vi "Rx-Maping Detail's.vi"(7 "Data Cluster In":T1, 8 "error in (no error)":errorcluster) -> (0 "error out":errorcluster, 5 "Data Cluster Out":T1)   [LabVIEW 2021, in "Test Panel.lvlib"]
doc: "<b>Note:</b> This VI was modified by the <b>Validate DQMH Module</b> tool to turn off automatic error handling."
uses:
  Test Panel.lvlib
  Module Data--cluster.ctl
  GUI Ctrl Data's--Cluster.ctl
  Rx-Mapping Data.ctl
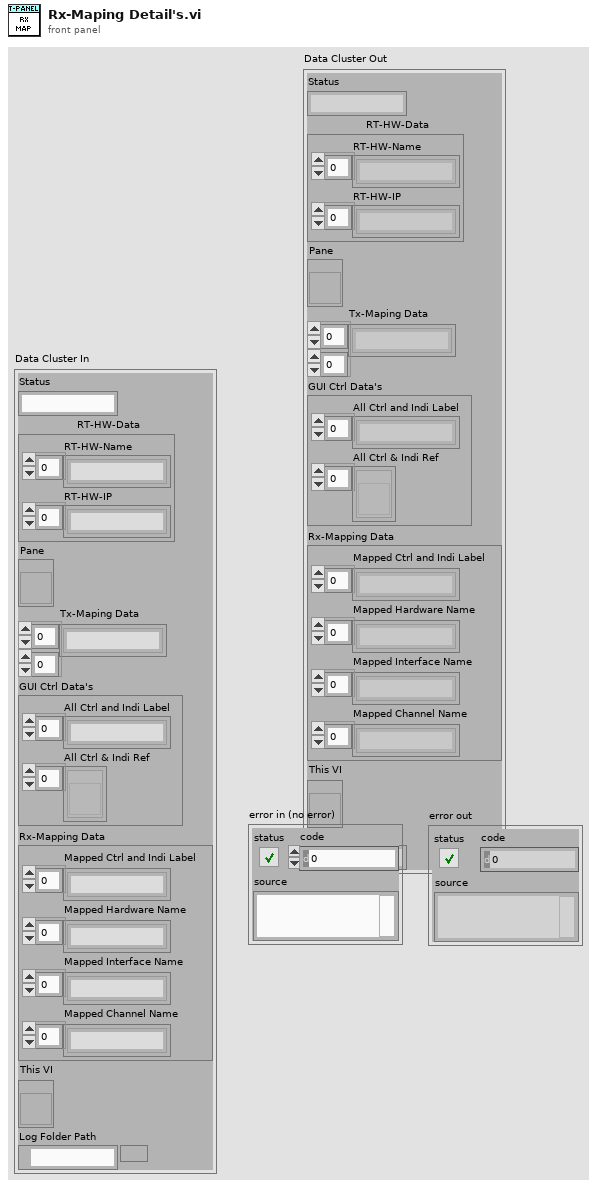
[diagram p1: front panel]
types:
  T1 = typedef "Test Panel.lvlib/Module Data--cluster.ctl" = cluster{"Status":string, "RT-HW-Data":cluster{"RT-HW-Name":string[], "RT-HW-IP":string[]}, "Pane":refnum<vi>, "Tx-Maping Data":string[][], "GUI Ctrl Data's":T2, "Rx-Mapping Data":T3, "This VI":refnum<vi>, "Log Folder Path":path}
  T2 = typedef "Test Panel.lvlib/GUI Ctrl Data's--Cluster.ctl" = cluster{"All Ctrl and Indi Label":string[], "All Ctrl & Indi Ref":refnum<vi>[]}
  T3 = typedef "Test Panel.lvlib/Rx-Mapping Data.ctl" = cluster{"Mapped Ctrl and Indi Label":string[], "Mapped Hardware Name":string[], "Mapped Interface Name":string[], "Mapped Channel Name":string[]}
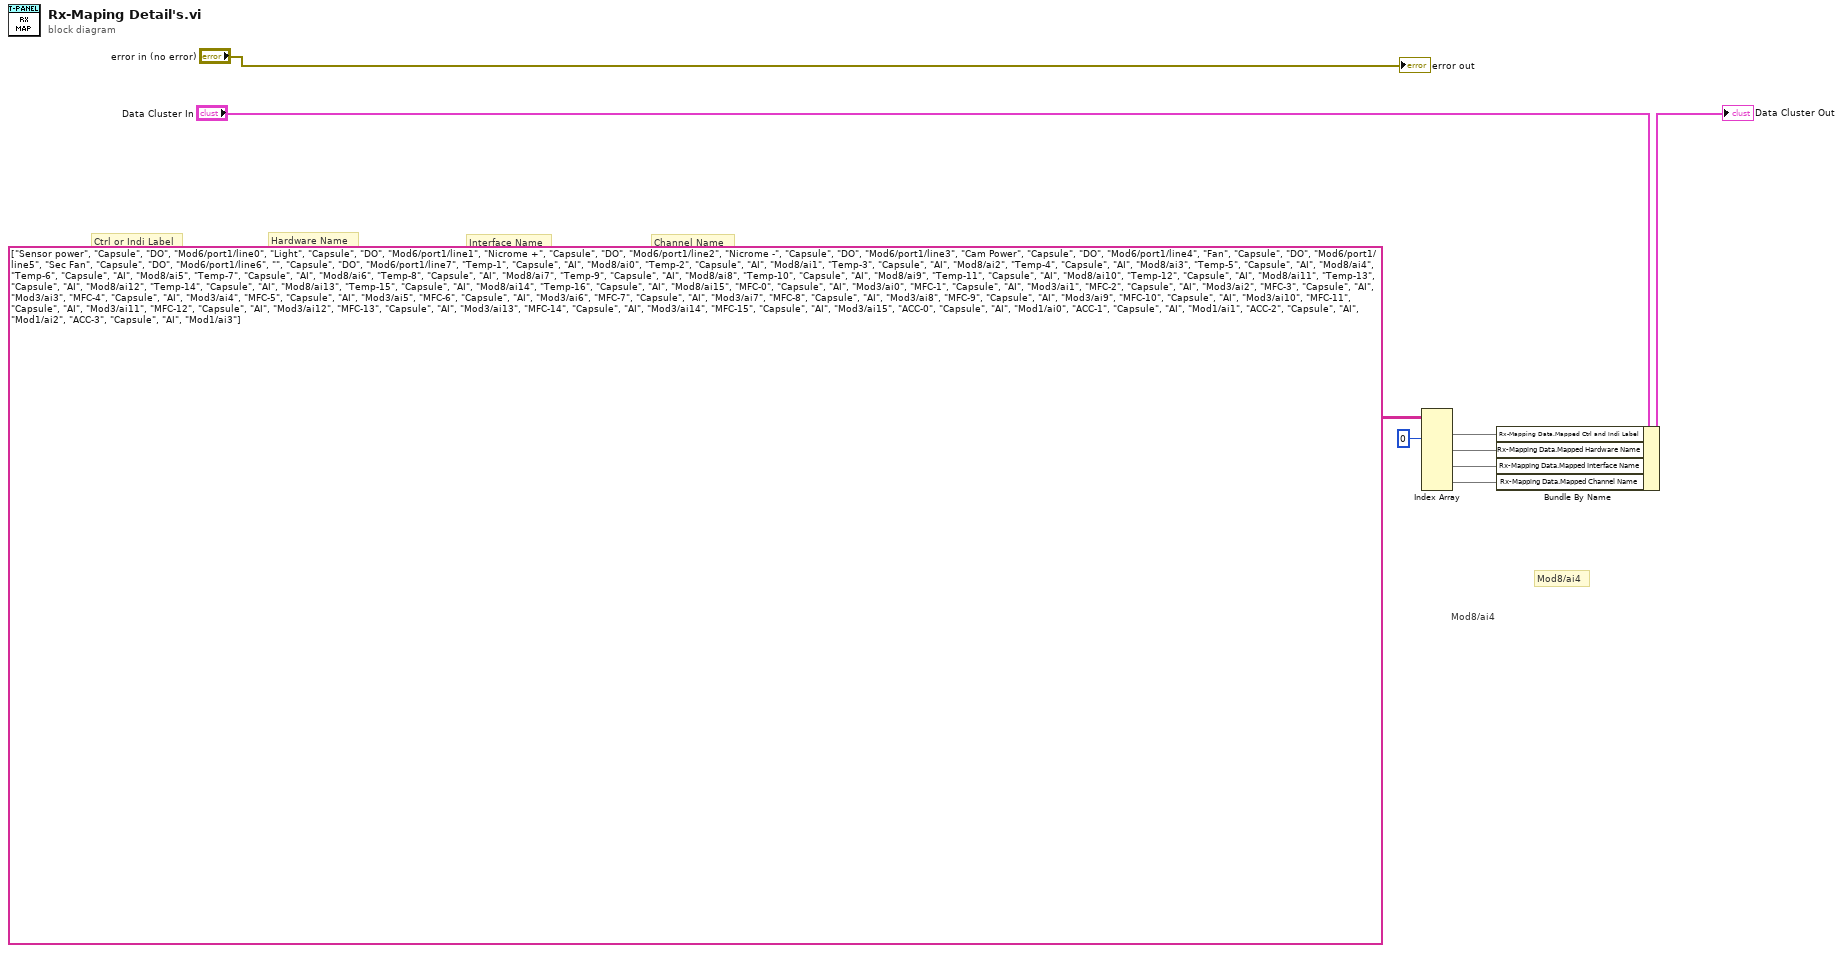
[diagram p0: block diagram]
diagram:
  # "Mod8/ai4"
  # "Mod8/ai4"
  # "Channel Name"
  # "Ctrl or Indi Label"
  # "Interface Name"
  # "Hardware Name"
  n1 = Index Array(array=string[][] [["Sensor power", "Capsule", "DO", "Mod6/port1/line0"], ["Light", "Capsule", "DO", "Mod6/port1/line1"], ["Nicrome +", "Capsule", "DO", "Mod6/port1/line2"], ["Nicrome -", "Capsule", "DO", "Mod6/port1/line3"], ["Cam Power", "Capsule", "DO", "Mod6/port1/line4"], ["Fan", "Capsule", "DO", "Mod6/port1/line5"], ["Sec Fan", "Capsule", "DO", "Mod6/port1/line6"], ["", "Capsule", "DO", "Mod6/port1/line7"], ["Temp-1", "Capsule", "AI", "Mod8/ai0"], ["Temp-2", "Capsule", "AI", "Mod8/ai1"], ["Temp-3", "Capsule", "AI", "Mod8/ai2"], ["Temp-4", "Capsule", "AI", "Mod8/ai3"], ["Temp-5", "Capsule", "AI", "Mod8/ai4"], ["Temp-6", "Capsule", "AI", "Mod8/ai5"], ["Temp-7", "Capsule", "AI", "Mod8/ai6"], ["Temp-8", "Capsule", "AI", "Mod8/ai7"], ["Temp-9", "Capsule", "AI", "Mod8/ai8"], ["Temp-10", "Capsule", "AI", "Mod8/ai9"], ["Temp-11", "Capsule", "AI", "Mod8/ai10"], ["Temp-12", "Capsule", "AI", "Mod8/ai11"], ["Temp-13", "Capsule", "AI", "Mod8/ai12"], ["Temp-14", "Capsule", "AI", "Mod8/ai13"], ["Temp-15", "Capsule", "AI", "Mod8/ai14"], ["Temp-16", "Capsule", "AI", "Mod8/ai15"], ["MFC-0", "Capsule", "AI", "Mod3/ai0"], ["MFC-1", "Capsule", "AI", "Mod3/ai1"], ["MFC-2", "Capsule", "AI", "Mod3/ai2"], ["MFC-3", "Capsule", "AI", "Mod3/ai3"], ["MFC-4", "Capsule", "AI", "Mod3/ai4"], ["MFC-5", "Capsule", "AI", "Mod3/ai5"], ["MFC-6", "Capsule", "AI", "Mod3/ai6"], ["MFC-7", "Capsule", "AI", "Mod3/ai7"], ["MFC-8", "Capsule", "AI", "Mod3/ai8"], ["MFC-9", "Capsule", "AI", "Mod3/ai9"], ["MFC-10", "Capsule", "AI", "Mod3/ai10"], ["MFC-11", "Capsule", "AI", "Mod3/ai11"], ["MFC-12", "Capsule", "AI", "Mod3/ai12"], ["MFC-13", "Capsule", "AI", "Mod3/ai13"], ["MFC-14", "Capsule", "AI", "Mod3/ai14"], ["MFC-15", "Capsule", "AI", "Mod3/ai15"], ["ACC-0", "Capsule", "AI", "Mod1/ai0"], ["ACC-1", "Capsule", "AI", "Mod1/ai1"], ["ACC-2", "Capsule", "AI", "Mod1/ai2"], ["ACC-3", "Capsule", "AI", "Mod1/ai3"]], index (col) #1=0 ("index (col)")) -> (element #1=w6:string[], element #2=w4:string[], element #3=w3:string[], element #4=w2:string[])  [unwired: 7 in]
  n2 = Bundle By Name(cluster="Data Cluster In", "Rx-Mapping Data.Mapped Ctrl and Indi Label"=w6, "Rx-Mapping Data.Mapped Hardware Name"=w4, "Rx-Mapping Data.Mapped Interface Name"=w3, "Rx-Mapping Data.Mapped Channel Name"=w2) -> (→"Data Cluster Out":T1)
  "error out" <- "error in (no error)"
